vi "MakeRunListGroups.vi"(7 "error in":errorcluster, 10 "WheelList":string[][](array[string])) -> (0 "error out":errorcluster, 1 "Runlist":i32[][](array[numeric]), 2 "SampleCount":i32, 3 "First Sample":i32)   [LabVIEW 2013]
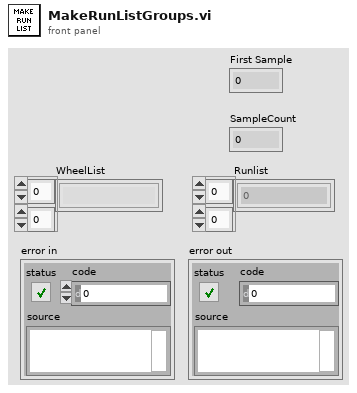
[diagram p1: front panel]
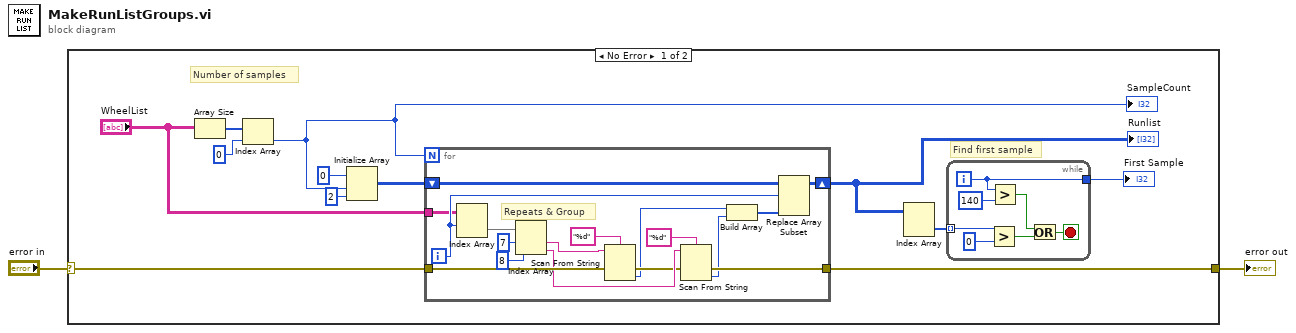
[diagram p0: block diagram]
diagram:
  n1 = case shown="No Error" "error in" {
    selector: "error in" -> [w8 w39]
    tunnel: [w7 w39] -> w1
    frame No Error {
      # "Find first sample"
      # "Number of samples"
      n2 = Array Size(array="WheelList") -> (size(s)=w14:i32[])
      n3 = Index Array(array=w14, index=0) -> (element=w10:i32)
      "SampleCount" <- w10
      n4 = Initialize Array(0 ("element"), w10, 2 ("dimension size")) -> (w11:i32[][])
      n5 = for {
        N: w10 -> [_]
        shift-right: [w38] -> w5
        shift-left: w11 -> [w32]
        tunnel: "WheelList" -> [w31]
        tunnel: w8 -> [w30]
        tunnel: [w26] -> w7
        i -> [w34]
        # "Repeats & Group"
        n6 = Index Array(array=w31, index (row)=w34) -> (element=w33:string[])  [unwired: 1 in]
        n7 = Index Array(array=w33, index #1=7 ("index"), index #2=8 ("index")) -> (element #1=w36:string, element #2=w28:string)
        n8 = Scan From String(format string="%d", input string=w36, error in=w30) -> (error out=w27:errorcluster, output 1=w25:i32)  [unwired: 1 in, 3 out]
        n9 = Scan From String(format string="%d", input string=w28, error in=w27) -> (error out=w26:errorcluster, output 1=w24:i32)  [unwired: 1 in, 3 out]
        n10 = Build Array(w25, w24) -> (w23:i32[])
        n11 = Replace Array Subset(array=w32, new element=w23, index (row)=w34) -> (w38:i32[][])  [unwired: 1 in]
      }
      "Runlist" <- w5
      n12 = Index Array(array=w5) -> (element=w4:i32[])  [unwired: 2 in]
      n13 = while {
        tunnel: w4 -> [w19] mode=indexing
        tunnel: [w17] -> w6
        i -> [w17]
        stop <- w18 stop-if-true
        n14 = Greater?(x=w19, y=0) -> (0:w20:bool)
        n15 = Greater?(x=w17, y=140) -> (0:w15:bool)
        n16 = Or(x=w15, y=w20) -> (x .or. y?=w18:bool)
      }
      "First Sample" <- w6
    }
    frame Error {
    }
  }
  "error out" <- w1
